vi "Get Project Conditional Disable Symbols.vi"(8 "error in (no error)":errorcluster {"code" format="Error %.0f"}, 9 "Project in":refnum<vi>) -> (0 "error out":errorcluster {"code" format="Error %.0f"}, 1 "Project out":refnum<vi>, 3 "Conditional Disable Symbols":string[][](array[string]))   [LabVIEW 2023, in "VIDoc Parsing.lvlib" / "Project Documentation.lvclass"]
uses:
  Project Documentation.lvclass
  Project Documentation.lvclass/Project Documentation.ctl
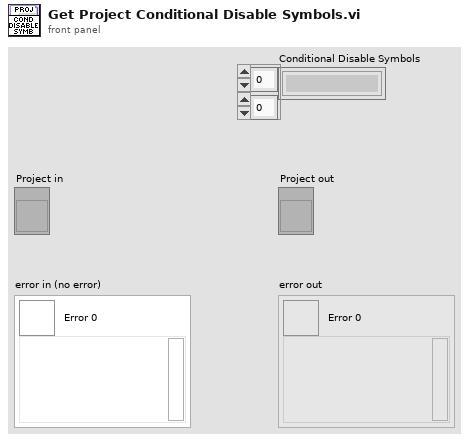
[diagram p1: front panel]
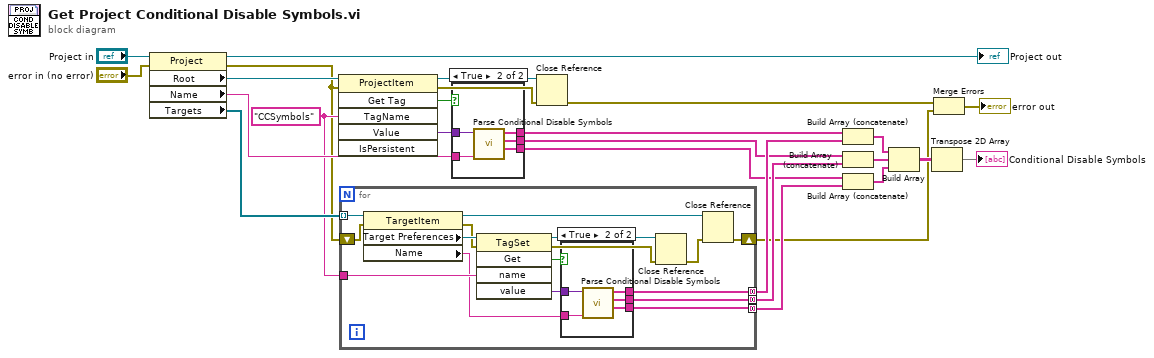
[diagram p0: block diagram]
diagram:
  w19 = "CCSymbols" ("Name")
  n1 = property class="Project"(reference="Project in", error in="error in (no error)") -> (reference out=→"Project out":refnum<vi>, error out=w17:errorcluster, "Root"=w25:refnum<vi>, "Name"=w22:string, "Targets"=w21:refnum<vi>[])
  n2 = invoke class="ProjectItem" method="Get Tag"(reference=w25, error in=w17, "TagName"=w19) -> (reference out=w20:refnum<vi>, error out=w18:errorcluster, "GetTag"=w23:bool, "Value"=w26:variant)  [unwired: 3 in, 2 out]
  n3 = for {
    tunnel: w21 -> [w42] mode=indexing
    tunnel: w19 -> [w40]
    tunnel: [w36] -> w15 mode=concatenating
    tunnel: [w35] -> w13 mode=concatenating
    tunnel: [w34] -> w11 mode=concatenating
    shift-right: [w28] -> w3
    shift-left: w17 -> [w27]
    n4 = property class="TargetItem"(reference=w42, error in=w27) -> (reference out=w30:refnum<vi>, error out=w32:errorcluster, "Target Preferences"=w41:refnum<vi>, "Name"=w37:string)
    n5 = invoke class="TagSet" method="Get"(reference=w41, error in=w32, "name"=w40) -> (reference out=w33:refnum<vi>, error out=w31:errorcluster, "Get"=w39:bool, "value"=w38:variant)  [unwired: 2 in, 1 out]
    n6 = case shown="True" w39 {
      tunnel: w38 -> [_ w45]
      tunnel: w37 -> [_ w47]
      tunnel: [_ w46] -> w35
      tunnel: [_ w44] -> w36
      tunnel: [_ w43] -> w34
      frame False {
      }
      frame True {
        n7 = call "Parse Conditional Disable Symbols.vi"("Target Name"=w47, "CCSymbols Value"=w45) -> ("Values"=w43:string[], "Symbols"=w46:string[], "Targets"=w44:string[])  [unwired: 7 in]
      }
    }
    n8 = Close Reference(reference=w33, error in (no error)=w31) -> (error out=w29:errorcluster)
    n9 = Close Reference(reference=w30, error in (no error)=w29) -> (error out=w28:errorcluster)
  }
  n10 = case shown="True" w23 {
    tunnel: w26 -> [_ w50]
    tunnel: w22 -> [_ w52]
    tunnel: [_ w51] -> w14
    tunnel: [_ w49] -> w16
    tunnel: [_ w48] -> w12
    frame False {
    }
    frame True {
      n11 = call "Parse Conditional Disable Symbols.vi"("Target Name"=w52, "CCSymbols Value"=w50) -> ("Values"=w48:string[], "Symbols"=w51:string[], "Targets"=w49:string[])  [unwired: 7 in]
    }
  }
  n12 = Close Reference(reference=w20, error in (no error)=w18) -> (error out=w4:errorcluster)
  n13 = Build Array (concatenate)(w16, w15) -> (w9:string[])
  n14 = Build Array (concatenate)(w14, w13) -> (w10:string[])
  n15 = Build Array (concatenate)(w12, w11) -> (w8:string[])
  n16 = Build Array(w9, w10, w8) -> (w7:string[][])
  n17 = Transpose 2D Array(2D array=w7) -> (transposed array=→"Conditional Disable Symbols":string[][])
  n18 = Merge Errors(w4, w3) -> (→"error out":errorcluster)
